vi "Util_Progress Close Progress Popup with Status.vi"(8 "error in (no error)":errorcluster) -> (0 "error out":errorcluster)   [LabVIEW 2013]
panel:
  out "appended path":path
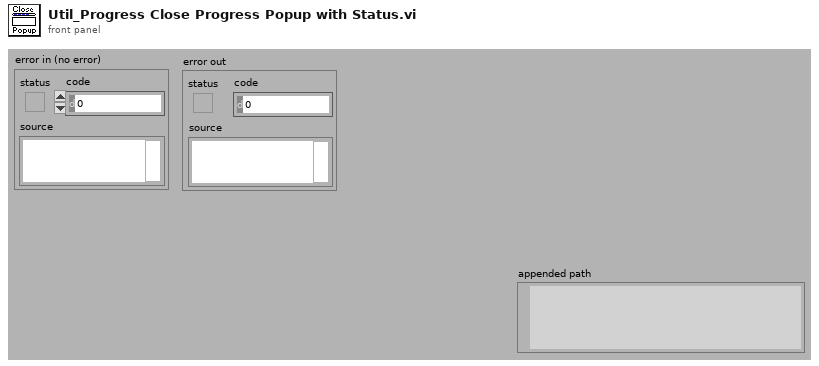
[diagram p1: front panel]
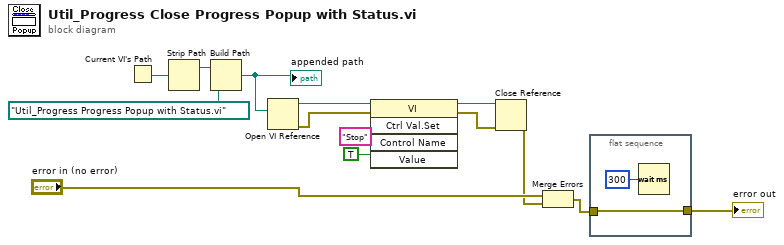
[diagram p0: block diagram]
diagram:
  n1 = Current VI's Path() -> (path=w14:path)
  n2 = Strip Path(path=w14) -> (stripped path=w13:path)  [unwired: 1 out]
  n3 = Build Path(base path=w13, name or relative path=path "Util_Progress Progress Popup with Status.vi" ("vi path")) -> (appended path=w11:path)
  "appended path" <- w11
  n4 = Open VI Reference(vi path=w11) -> (vi reference=w10:refnum<vi>, error out=w5:errorcluster)  [unwired: 1 in, 4 out]
  n5 = invoke class="VI" method="Ctrl Val.Set"(reference=w10, error in=w5, "Control Name"="Stop", "Value"=TRUE) -> (reference out=w8:refnum<vi>, error out=w9:errorcluster)  [unwired: 1 in, 3 out]
  n6 = Close Reference(reference=w8, error in (no error)=w9) -> (error out=w3:errorcluster)
  n7 = Merge Errors("error in (no error)", w3) -> (w2:errorcluster)
  n8 = flat-sequence {
    tunnel: w2 -> [w16]
    tunnel: [w16] -> w1
    frame #0 {
      n9 = Wait (ms)(milliseconds to wait=u32 300) -> ()  [unwired: 1 out]
    }
  }
  "error out" <- w1
